vi "Config Continuous.vi"(7 "Reset (true)":bool=TRUE, 8 "error in":errorcluster, 9 "Total (0)":i32 min=0 max=99999999, 10 "Interval (0)":dbl min=0.0 max=99999999.0 step=0.1 format="%#_10f", 11 "VISA resource name":refnum<visa-resource-name>) -> (0 "error out":errorcluster, 3 "VISA resource name out":refnum<visa-resource-name>)   [LabVIEW 2018, in "Andeen-Hagerling 2700.lvlib"]
doc: "This VI configures the bridge to take continuous measurements. Specifically, the continuous total and continuous interval parameters are set. Additionally, the continous count variable is zeroed when <b>Continuous Reset</b> is set to true."
uses:
  Andeen-Hagerling 2700.lvlib
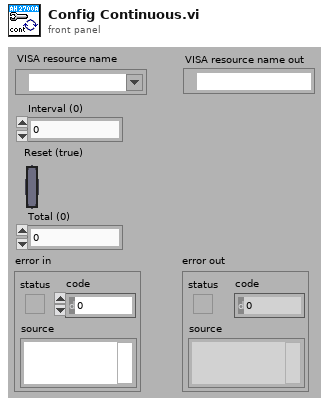
[diagram p1: front panel]
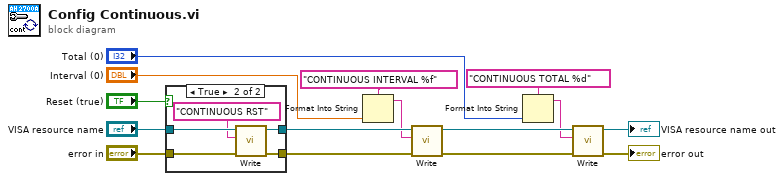
[diagram p0: block diagram]
diagram:
  n1 = case shown="True" "Reset (true)" {
    tunnel: "VISA resource name" -> [w17 w22]
    tunnel: "error in" -> [w16 w21]
    tunnel: [w16 w20] -> w13
    tunnel: [w17 w19] -> w14
    frame False {
    }
    frame True {
      n2 = call "Write.vi"("error in"=w21, "command"="CONTINUOUS RST", "VISA resource name"=w22) -> ("error out"=w20:errorcluster, "VISA resource name out"=w19:refnum<visa-resource-name>)  [unwired: 7 in]
    }
  }
  n3 = Format Into String(format string="CONTINUOUS INTERVAL %f", "Interval (0)") -> (resulting string=w12:string)  [unwired: 2 in, 1 out]
  n4 = call "Write.vi"("error in"=w13, "command"=w12, "VISA resource name"=w14) -> ("error out"=w9:errorcluster, "VISA resource name out"=w10:refnum<visa-resource-name>)  [unwired: 7 in]
  n5 = Format Into String(format string="CONTINUOUS TOTAL %d", "Total (0)") -> (resulting string=w8:string)  [unwired: 2 in, 1 out]
  n6 = call "Write.vi"("error in"=w9, "command"=w8, "VISA resource name"=w10) -> ("error out"=→"error out":errorcluster, "VISA resource name out"=→"VISA resource name out":refnum<visa-resource-name>)  [unwired: 7 in]
